vi "ParseResponse.vi"(6 "Command":string, 8 "error in (no error)":errorcluster, 11 "Response":string) -> (0 "error out":errorcluster, 3 "val":string, 4 "OK":bool, 5 "BD":i32)   [LabVIEW 2020, in "CAEN PSM.lvlib"]
uses:
  CAEN PSM.lvlib
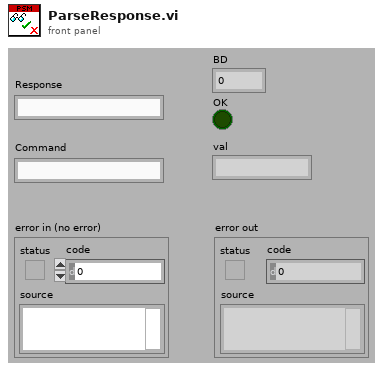
[diagram p1: front panel]
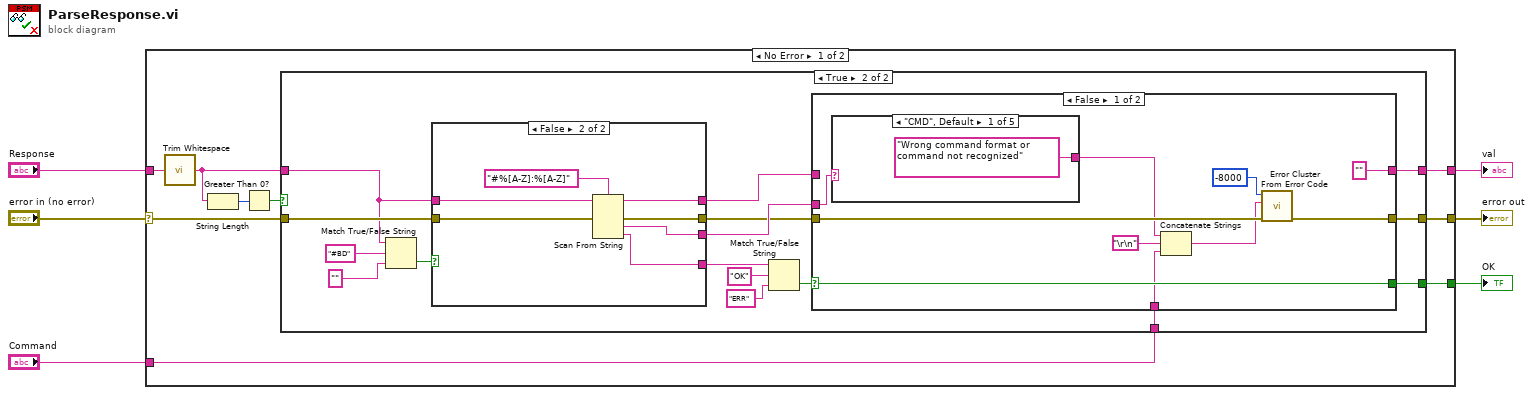
[diagram p0: block diagram]
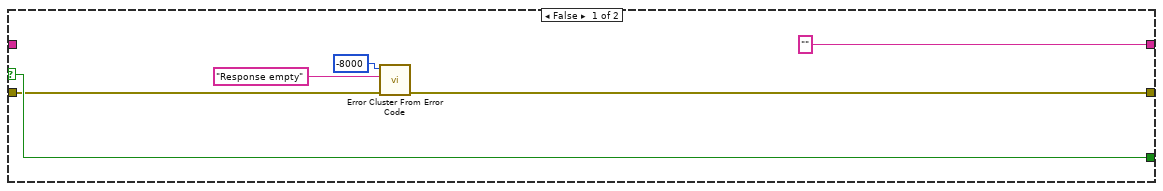
[diagram p2: hidden frame]
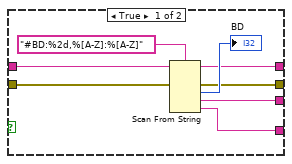
[diagram p3: hidden frame]
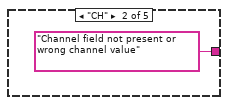
[diagram p4: hidden frame]
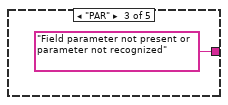
[diagram p5: hidden frame]
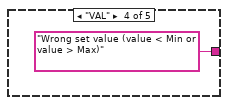
[diagram p6: hidden frame]
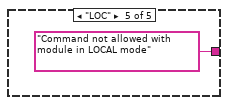
[diagram p7: hidden frame]
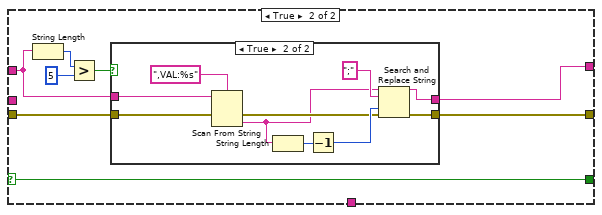
[diagram p8: hidden frame]
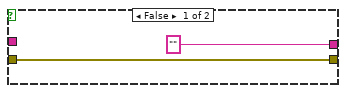
[diagram p9: hidden frame]
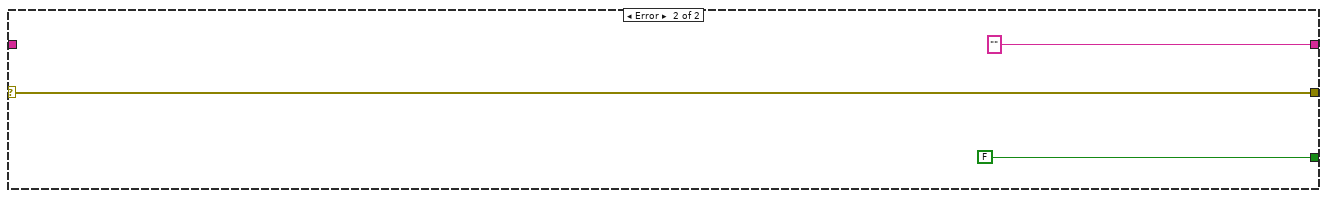
[diagram p10: hidden frame]
diagram:
  n1 = case shown="No Error" "error in (no error)" {
    selector: "error in (no error)" -> [w8 w90]
    tunnel: [w15 ""] -> w6
    tunnel: [w14 w90] -> w5
    tunnel: [w13 FALSE] -> w4
    tunnel: "Response" -> [w10 _]
    tunnel: "Command" -> [w7 _]
    frame No Error {
      n2 = call "Trim Whitespace.vi"("string"=w10) -> ("trimmed string"=w9:string)  [unwired: 1 in]
      n3 = String Length(string=w9) -> (length=w12:i32)
      n4 = Greater Than 0?(x=w12) -> (x > 0?=w11:bool)
      n5 = case shown="True" w11 {
        selector: w11 -> [w21 _]
        tunnel: w8 -> [w19 w37]
        tunnel: ["" w33] -> w15
        tunnel: [w20 w32] -> w14
        tunnel: [w21 w31] -> w13
        tunnel: w9 -> [_ w24]
        tunnel: w7 -> [_ w22]
        frame False {
          n6 = call "Error Cluster From Error Code.vi"("error in (no error)"=w19, "error message (\"\")"="Response empty" ("error message (\"\")"), "error code (0)"=-8000) -> ("error out"=w20:errorcluster)  [unwired: 6 in]
        }
        frame True {
          n7 = Match True/False String(2:"" ("false string"), 3:"#BD" ("true string"), 4:w24) -> (0:w26:bool)  [unwired: 1 out]
          n8 = case shown="False" w26 {
            tunnel: w37 -> [w44 w51]
            tunnel: [w42 w46] -> w30
            tunnel: [w41 w47] -> w29
            tunnel: [w40 w50] -> w28
            tunnel: [w39 w49] -> w27
            tunnel: w24 -> [w38 w48]
            frame True {
              n9 = Scan From String(format string="#BD:%2d,%[A-Z]:%[A-Z]", input string=w38, error in=w44) -> (remaining string=w40:string, error out=w39:errorcluster, output 1=→"BD":i32, output 2=w41:string, output 3=w42:string)  [unwired: 4 in, 1 out]
            }
            frame False {
              n10 = Scan From String(format string="#%[A-Z]:%[A-Z]", input string=w48, error in=w51) -> (remaining string=w50:string, error out=w49:errorcluster, output 1=w47:string, output 2=w46:string)  [unwired: 3 in, 1 out]
            }
          }
          n11 = Match True/False String(2:"ERR" ("false string"), 3:"OK" ("true string"), 4:w30) -> (0:w34:bool)  [unwired: 1 out]
          n12 = case shown="False" w34 {
            selector: w34 -> [w57 w73]
            tunnel: w29 -> [w62 _]
            tunnel: w28 -> [_ w72]
            tunnel: ["" w68] -> w33
            tunnel: w27 -> [w59 w75]
            tunnel: [w60 w74] -> w32
            tunnel: [w57 w73] -> w31
            tunnel: w22 -> [w53 _]
            frame False {
              n13 = case shown="\"CMD\", Default" w62 {
                tunnel: ["Wrong command format or command not recognized" "Channel field not present or wrong channel value" "Field parameter not present or parameter not recognized" "Wrong set value (value < Min or value > Max)" "Command not allowed with module in LOCAL mode"] -> w55
                frame "CMD", Default {
                }
                frame "CH" {
                }
                frame "PAR" {
                }
                frame "VAL" {
                }
                frame "LOC" {
                }
              }
              n14 = Concatenate Strings(w55, "\r\n", w53) -> (w54:string)
              n15 = call "Error Cluster From Error Code.vi"("error in (no error)"=w59, "error message (\"\")"=w54, "error code (0)"=-8000) -> ("error out"=w60:errorcluster)  [unwired: 6 in]
            }
            frame True {
              n16 = String Length(string=w72) -> (length=w70:i32)
              n17 = Greater?(x=w70, y=5) -> (0:w71:bool)
              n18 = case shown="True" w71 {
                tunnel: ["" w78] -> w68
                tunnel: w75 -> [w76 w86]
                tunnel: [w76 w79] -> w74
                tunnel: w72 -> [_ w85]
                frame False {
                }
                frame True {
                  n19 = Scan From String(format string=",VAL:%s", input string=w85, error in=w86) -> (error out=w81:errorcluster, output 1=w80:string)  [unwired: 2 in, 2 out]
                  n20 = String Length(string=w80) -> (length=w84:i32)
                  n21 = Decrement(x=w84) -> (x-1=w83:i32)
                  n22 = Search and Replace String(input string=w80, search string=";", offset=w83, error in=w81) -> (result string=w78:string, error out=w79:errorcluster)  [unwired: 4 in, 2 out]
                }
              }
            }
          }
        }
      }
    }
    frame Error {
    }
  }
  "error out" <- w5
  "val" <- w6
  "OK" <- w4
